vi "Generate Config Changed User Event.vi"(8 "error in (no error)":errorcluster) -> (0 "error out":errorcluster)   [LabVIEW 2015, in "System Config.lvclass"]
uses:
  System Config.lvclass
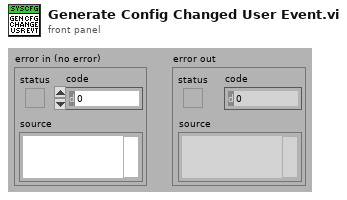
[diagram p1: front panel]
types:
  T1 = typedef "System Config.lvclass/ClassAttributes.ctl" = cluster{"Config":cluster{"Logging":cluster{"Log Files Directory":path, "Max Lines Per Log File":i32}, "Settings":T2}, "Core":cluster{"Config Directory":path, "Name":string, "Config Changed":refnum<user-event>}}
  T2 = typedef "System Config.lvclass/Settings.ctl" = cluster{"Dummy":dbl}
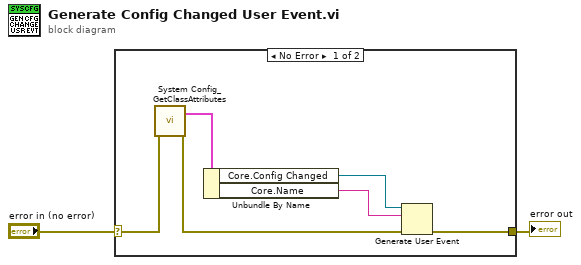
[diagram p0: block diagram]
diagram:
  n1 = case shown="No Error" "error in (no error)" {
    selector: "error in (no error)" -> [w8 w9]
    tunnel: [w4 w9] -> w1
    frame No Error {
      n2 = call "System Config_GetClassAttributes.vi"("error in (no error)"=w8) -> ("error out"=w5:errorcluster, "class attributes"=w7:T1)  [unwired: 7 in, 2 out]
      n3 = Unbundle By Name(w7) -> ("Core.Config Changed"=w6:refnum<user-event>, "Core.Name"=w3:string)
      n4 = Generate User Event(user event=w6, event data cluster=w3, error in=w5) -> (error out=w4:errorcluster)  [unwired: 1 in, 1 out]
    }
    frame Error {
    }
  }
  "error out" <- w1
